vi "Build Tx Command Word.vi"(8 "error in (no error)":errorcluster, 11 "Async RT-RT Message in":refnum<class "Async RT-RT Message.lvclass">) -> (0 "error out":errorcluster, 2 "Tx Command Word":u16)   [LabVIEW 2020, in "BCI-1553 API.lvlib" / "Async RT-RT Message.lvclass"]
doc: "<DO NOT CALL>\n\nSets up the message command word. This is the 1553 protocol word that will preface any data transactions required by this bus controller."
uses:
  Async RT-RT Message.lvclass
  TypeDefs/Command Type.ctl
  Async RT-RT Message.lvclass/Async RT-RT Message.ctl
  BCI-1553 API.lvlib
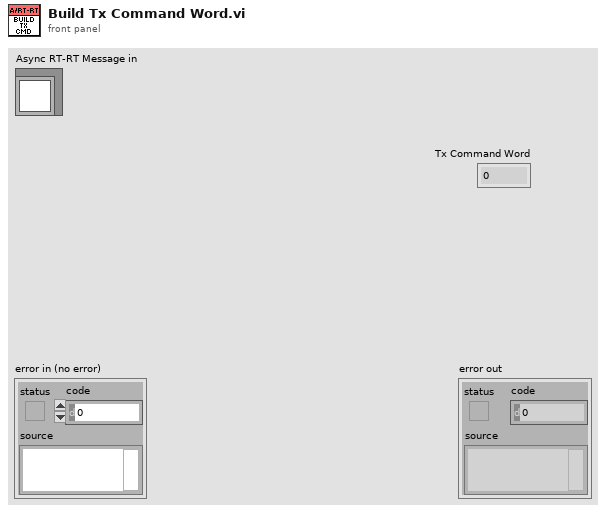
[diagram p1: front panel]
types:
  T1 = typedef "BCI-1553 API.lvlib/Command Type.ctl" = enum16{"Transmit", "Receive"}
  T2 = typedef "BCI-1553 API.lvlib/Command SubAddress.ctl" = enum16{"Mode Code", "1", "2", "3", "4", "5", "6", "7", "8", "9", "10", "11", "12", "13", "14", "15", "16", "17", "18", "19", "20", "21", "22", "23", "24", "25", "26", "27", "28", "29", "30"}
  T3 = typedef "BCI-1553 API.lvlib/Command Word Count.ctl" = enum16{"1", "2", "3", "4", "5", "6", "7", "8", "9", "10", "11", "12", "13", "14", "15", "16", "17", "18", "19", "20", "21", "22", "23", "24", "25", "26", "27", "28", "29", "30", "31", "32"}
  T4 = typedef "BCI-1553 API.lvlib/Command Terminal Address.ctl" = enum16{"0", "1", "2", "3", "4", "5", "6", "7", "8", "9", "10", "11", "12", "13", "14", "15", "16", "17", "18", "19", "20", "21", "22", "23", "24", "25", "26", "27", "28", "29", "30", "Broadcast"}
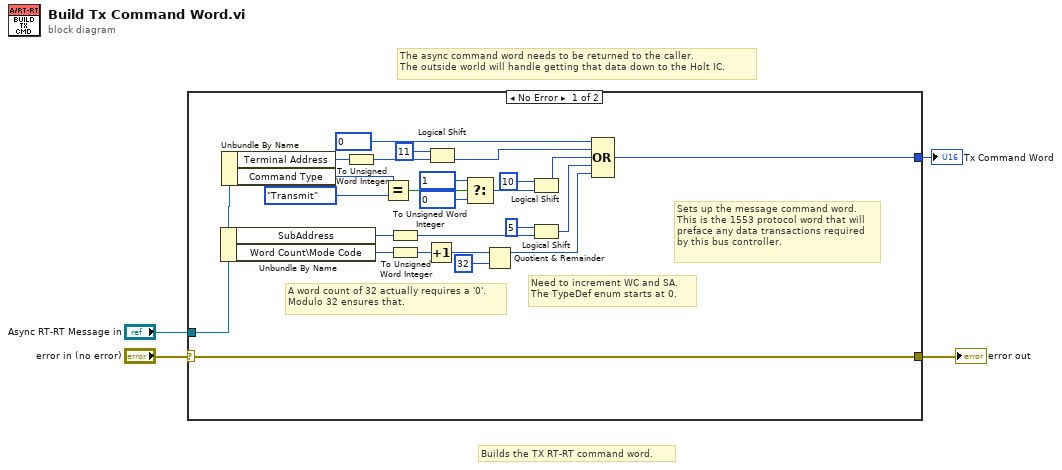
[diagram p0: block diagram]
diagram:
  # "Builds the TX RT-RT command word."
  # "The async command word needs to be returned to the caller.\nThe outside world will handle getting that data down to the Holt IC."
  n1 = case shown="No Error" "error in (no error)" {
    selector: "error in (no error)" -> [w29 w30]
    tunnel: [w29 w30] -> w2
    tunnel: "Async RT-RT Message in" -> [w23 _]
    tunnel: [w10 _] -> w1
    frame No Error {
      # "Need to increment WC and SA.\nThe TypeDef enum starts at 0."
      # "Sets up the message command word.\nThis is the 1553 protocol word that will\npreface any data transactions required\nby this bus controller."
      # "A word count of 32 actually requires a '0'.\nModulo 32 ensures that."
      n2 = Unbundle By Name(w23) -> ("SubAddress"=w15:T2, "Word Count\\Mode Code"=w11:T3)
      n3 = Unbundle By Name(w23) -> ("Terminal Address"=w27:T4, "Command Type"=w22:T1)
      n4 = To Unsigned Word Integer(number=w27) -> (unsigned 16bit integer=w7:u16)
      n5 = Equal?(x=w22, y=Command_Type."Transmit" ("RT-RT Async Message Config.Tx Command Config.Command Type")) -> (x = y?=w21:bool)
      n6 = To Unsigned Word Integer(number=w15) -> (unsigned 16bit integer=w6:u16)
      n7 = To Unsigned Word Integer(number=w11) -> (unsigned 16bit integer=w8:u16)
      n8 = Increment(x=w8) -> (x+1=w5:u16)
      n9 = Logical Shift(y=i16 11, x=w7) -> (x << y=w26:u16)
      n10 = Select(t=u16 1, s=w21, f=u16 0) -> (s? t:f=w18:u16)
      n11 = Quotient & Remainder(x=w5, y=u16 32) -> (x-y*floor(x/y)=w13:u16)  [unwired: 1 out]
      n12 = Logical Shift(y=i16 10, x=w18) -> (x << y=w17:u16)
      n13 = Logical Shift(y=i16 5, x=w6) -> (x << y=w14:u16)
      n14 = Compound Arithmetic op=OR(u16 0, w26, w17, w14, w13) -> (w10:u16)
    }
    frame Error {
    }
  }
  "error out" <- w2
  "Tx Command Word" <- w1
